vi "Control Panel Initialization Message.vi"(8 "error in (no error)":errorcluster, 10 "Resource":variant, 11 "LC Parser in":refnum<class "LC Parser.lvclass">) -> (0 "error out":errorcluster, 2 "Message":T1, 3 "LC Parser out":refnum<class "LC Parser.lvclass">)   [LabVIEW 2020, in "RxnRover.lvlib" / "LC Parser.lvclass"]
doc: "Method to generate the initial message to send to a Controller's Control Panel."
uses:
  LC Parser.lvclass
  <userlib>/RxnRover/DynamicReentrant/src/Type Defs/Message.ctl
  <userlib>/RxnRover/DynamicReentrant/Dynamic Reentrant.lvlib
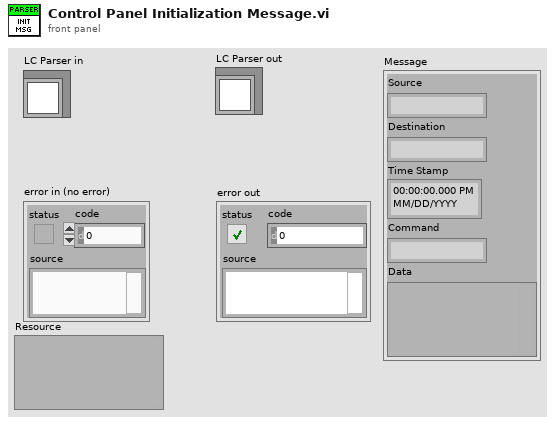
[diagram p1: front panel]
types:
  T1 = typedef "Dynamic Reentrant.lvlib/Message.ctl" = cluster{"Source":string, "Destination":string, "Time Stamp":timestamp, "Command":string, "Data":variant}
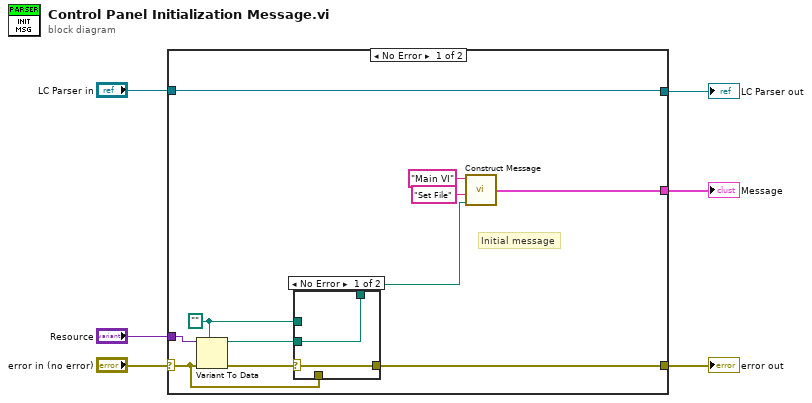
[diagram p0: block diagram]
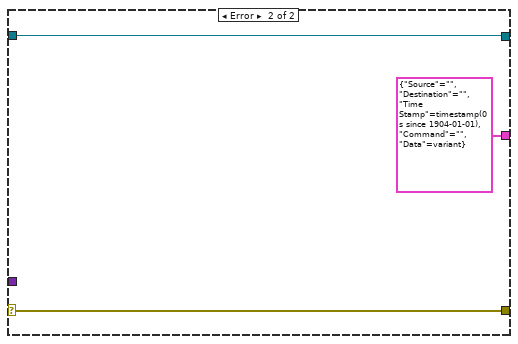
[diagram p3: hidden frame]
diagram:
  n1 = case shown="No Error" "error in (no error)" {
    selector: "error in (no error)" -> [w8 w24]
    tunnel: [w17 w23] -> w4
    tunnel: "LC Parser in" -> [w17 w23]
    tunnel: [w11 w24] -> w6
    tunnel: [w14 T1 {"Source"="", "Destination"="", "Time Stamp"=timestamp(0 s since 1904-01-01), "Command"="", "Data"=variant} ("output cluster")] -> w5
    tunnel: "Resource" -> [w13 _]
    frame No Error {
      w10 = path ""
      # "Initial message"
      n2 = Variant To Data(error in=w8, type=w10, Variant=w13) -> (data=w9:path, error out=w12:errorcluster)
      n3 = case shown="No Error" w12 {
        selector: w12 -> [w18 _]
        tunnel: w10 -> [_ w21]
        tunnel: w9 -> [w19 _]
        tunnel: [w19 w21] -> w7
        tunnel: [w18 w20] -> w11
        tunnel: w8 -> [_ w20]
        frame No Error {
        }
        frame Error {
        }
      }
      n4 = call <userlib>:"Construct Message.vi"("Data"=w7, "Command"="Set File", "Source"="Main VI") -> ("Message Cluster"=w14:T1)  [unwired: 3 in]
    }
    frame Error {
    }
  }
  "LC Parser out" <- w4
  "error out" <- w6
  "Message" <- w5
